vi "Find Diameter of Polygon.vi"(0 "Min Lat":dbl, 5 "Min Lon":dbl, 7 "Max Lat":dbl, 9 "Max Lon":dbl, 11 "Error In":errorcluster) -> (4 "Distance (km)":dbl, 15 "Error Out":errorcluster)   [LabVIEW 2014]
uses:
  Lat Long Conversion/Controls/PointLatLon.ctl
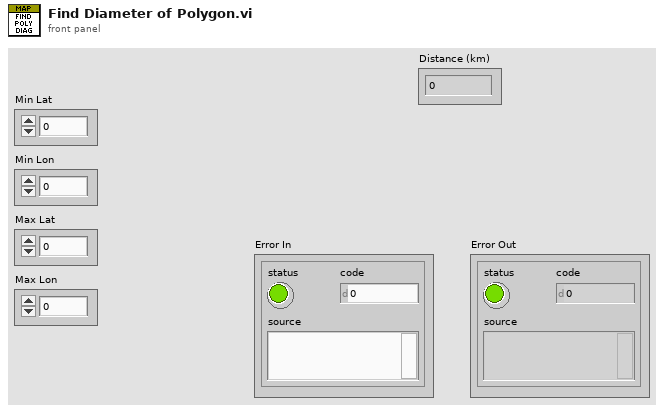
[diagram p1: front panel]
types:
  T1 = typedef "PointLatLon.ctl" = cluster{"Longitude":dbl, "Latitude":dbl}
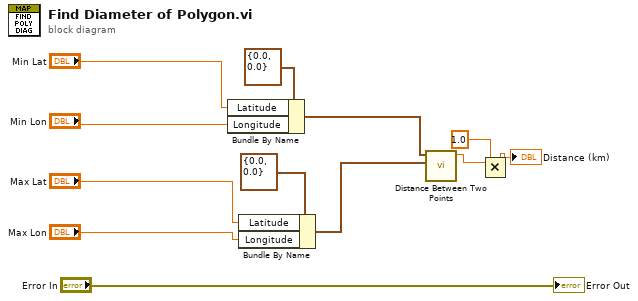
[diagram p0: block diagram]
diagram:
  n1 = Bundle By Name(cluster=T1 {"Longitude"=0.0, "Latitude"=0.0} ("Origin Point"), "Latitude"="Min Lat", "Longitude"="Min Lon") -> (w9:T1)
  n2 = Bundle By Name(cluster=T1 {"Longitude"=0.0, "Latitude"=0.0} ("Origin Point"), "Latitude"="Max Lat", "Longitude"="Max Lon") -> (w5:T1)
  n3 = call "Distance Between Two Points.vi"("Point 2"=w5, "Point 1"=w9) -> ("Distance (km)"=w3:dbl)  [unwired: 9 in]
  n4 = Multiply(x=w3, y=1.0) -> (x*y=→"Distance (km)":dbl)
  "Error Out" <- "Error In"
